vi "GetGlobalDefaultConfiguration.vi"(3 "Read defaults?":bool) -> ()   [LabVIEW 2018]
uses:
  QC_MeasurementSetup.vi
  InstrControl/InstrumentSetup.vi
  InstrControl/InstrControl.lvclass
panel:
  out "Configuration File Striptest":path
  out "Configuration File Cis":path
  out "Configuration File Stability":path
  out "Configuration File CV":path
  out "Configuration File IV":path
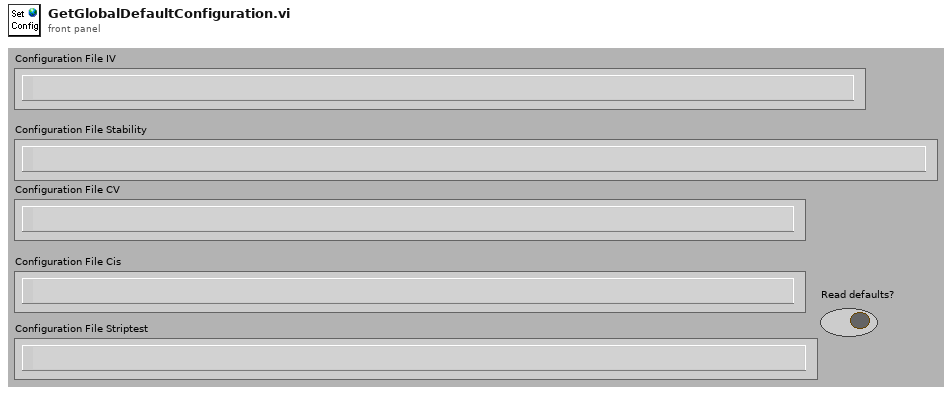
[diagram p1: front panel]
types:
  T1 = cluster{"Supply":refnum<class "SupplyControl.lvclass">, "Arduino":refnum<class "ArduinoControl.lvclass">, "Measurement switch":refnum<class "Switching.lvclass">, "Initial Voltage [V]":dbl, "Final Voltage [V]":dbl, "Step Size [V]":dbl, "Step Interval [s]":i32, "Number Of Steps":u32, "Ramp down steps [V]":dbl, "Ramp down Interval [s]":i32, "hold steps":i32, "Set Current Limit?":bool, "Current Limit [µA]":dbl, "Temperature Readout":enum16{"Read Arduino", "Enter manually"}, "Supply Name":string, "V_breakdown Limit [V]":dbl, "Measurement switch used?":bool}
  T2 = cluster{"Supply":refnum<class "SupplyControl.lvclass">, "LCR":refnum<class "LCRControl.lvclass">, "Arduino":refnum<class "ArduinoControl.lvclass">, "Measurement switch":refnum<class "Switching.lvclass">, "Initial Voltage [V]":dbl, "Final Voltage [V]":dbl, "Step Size [V]":dbl, "Step Interval [s]":i32, "Number Of Steps":u32, "Ramp down steps [V]":dbl, "Ramp down Interval [s]":i32, "Set Current Limit?":bool, "Current Limit [µA]":dbl, "Temperature Readout":enum16{"Read Arduino", "Enter manually"}, "Supply Name":string, "LCR Name":string, "V_depletion Limit [V]":dbl, "Measurement switch used?":bool}
  T3 = cluster{"RC Configuration":u16, "AC amplitude [V]":dbl, "AC frequency [Hz]":i32, "HP 4284A Configurations":cluster{"Consider OC":bool, "Consider SC":bool}}
  T4 = cluster{"Supply":refnum<class "SupplyControl.lvclass">, "DMM":refnum<class "MultimeterControl.lvclass">, "DUT switch":refnum<class "Switching.lvclass">, "Arduino":refnum<class "ArduinoControl.lvclass">, "Measurement switch":refnum<class "Switching.lvclass">, "Voltage [V]":dbl, "Measurement Interval [s]":i32, "Test Duration":u32, "Ramp up steps [V]":dbl, "Ramp up Interval [s]":u32, "Ramp down steps [V]":dbl, "Ramp down Interval [s]":i32, "Set Current Limit?":bool, "Current Limit [µA]":dbl, "Temperature Readout":enum16{"Read Arduino", "Enter manually"}, "Supply Name":string, "DMM Name":string, "Maximum current fluctuation [%]":dbl, "Measurement switch used?":bool, "DUT switch used?":bool}
  T5 = cluster{"Supply":refnum<class "SupplyControl.lvclass">, "LCR":refnum<class "LCRControl.lvclass">, "Arduino":refnum<class "ArduinoControl.lvclass">, "Measurement switch":refnum<class "Switching.lvclass">, "Initial Voltage [V]":dbl, "Final Voltage [V]":dbl, "Step Size [V]":dbl, "Step Interval [s]":i32, "Number Of Steps":u32, "AC frequency [Hz]":i32, "RC Configuration":u16, "AC amplitude [V]":dbl, "Ramp down steps [V]":dbl, "Ramp down Interval [s]":i32, "Set Current Limit?":bool, "Current Limit [µA]":dbl, "Temperature Readout":enum16{"Read Arduino", "Enter manually"}, "Supply Name":string, "LCR Name":string, "C_is Limit [pF/cm]":dbl, "Measurement switch used?":bool}
  T6 = cluster{"Bias Supply":refnum<class "SupplyControl.lvclass">, "SMU":refnum<class "SupplyControl.lvclass">, "LCR":refnum<class "LCRControl.lvclass">, "ProbeStation":refnum<class "ProbeStationControl.lvclass">, "Arduino":refnum<class "ArduinoControl.lvclass">, "Measurement switch":refnum<class "Switching.lvclass">, "Probe Card Channels":i32, "Bias Voltage [V]":dbl, "First strip":i32, "Last strip":i32, "Base Voltage [V]":dbl, "Base Ramp Step [V]":dbl, "Base Ramp Interval [ms]":u32, "High Voltage [V]":dbl, "High Ramp Step [V]":dbl, "High Ramp Interval [ms]":u32, "AC frequency [Hz]":i32, "AC amplitude [V]":dbl, "RC Configuration":u16, "Single Needle":bool, "Temperature Readout":enum16{"Read Arduino", "Enter manually"}, "Fraction of good strips [%]":dbl, "Measurement switch used?":bool, "Matrix X Channels":cluster{"Mux1 C1":i32, "Mux1 C2":i32, "Mux2 C1":i32, "Mux2 C2":i32}, "Pinholes Y/N":bool, "Capacitance Y/N":bool, "Resistance Y/N":bool, "Bias Supply Name":string, "SMU Name":string, "LCR Name":string}
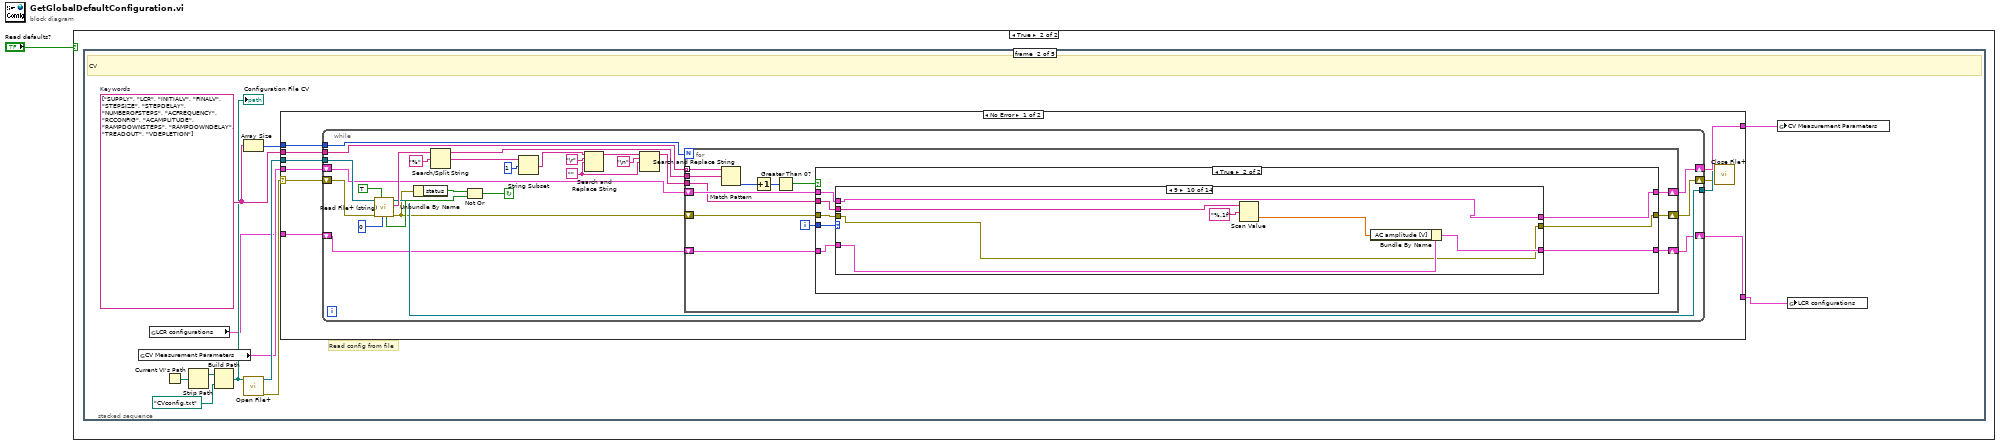
[diagram p0: block diagram]
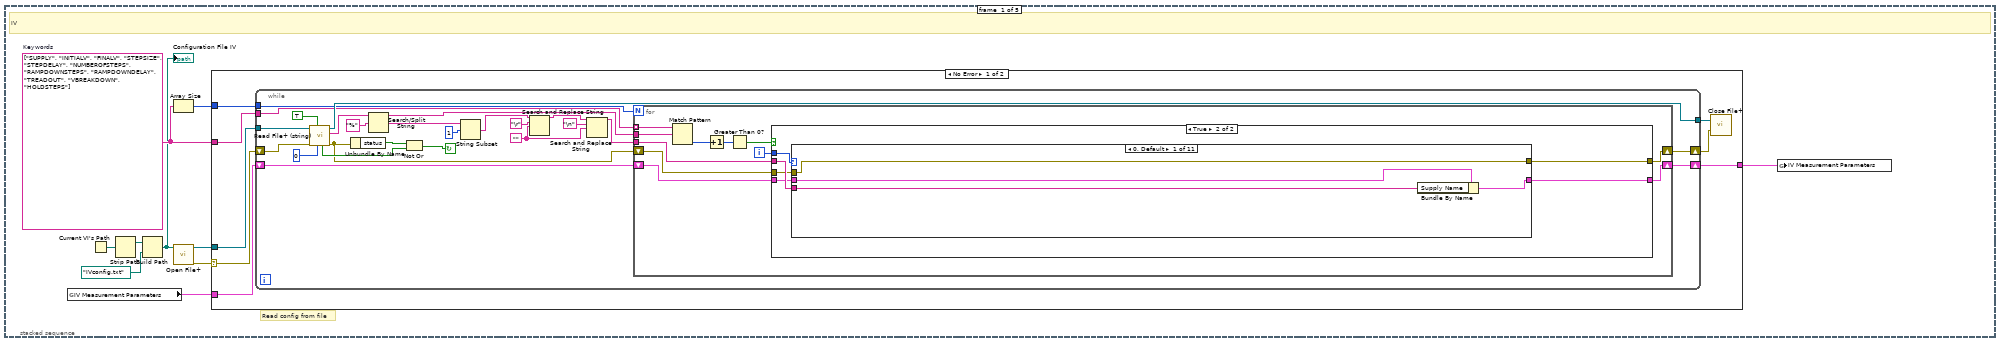
[diagram p3: hidden frame]
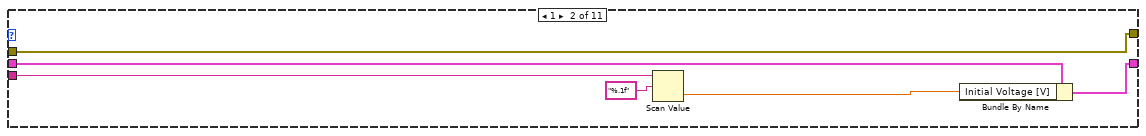
[diagram p5: hidden frame]
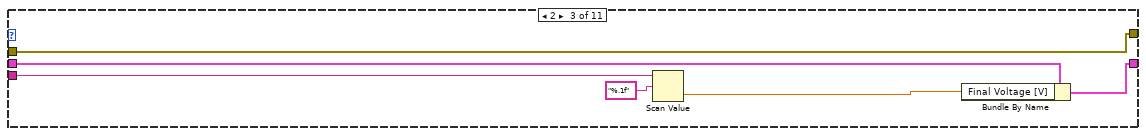
[diagram p6: hidden frame]
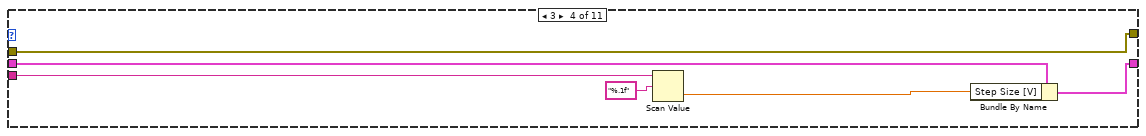
[diagram p7: hidden frame]
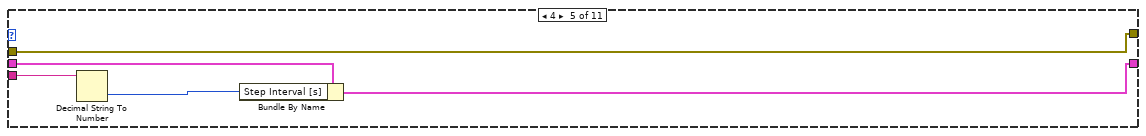
[diagram p8: hidden frame]
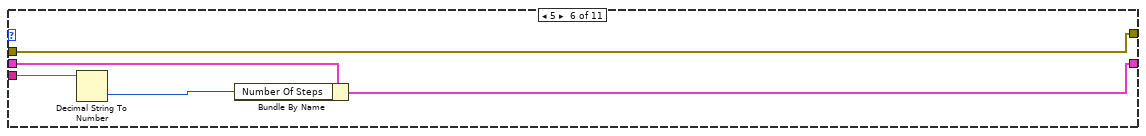
[diagram p9: hidden frame]
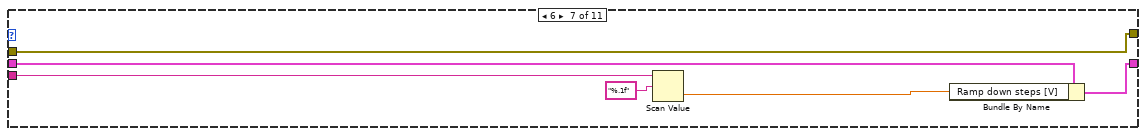
[diagram p10: hidden frame]
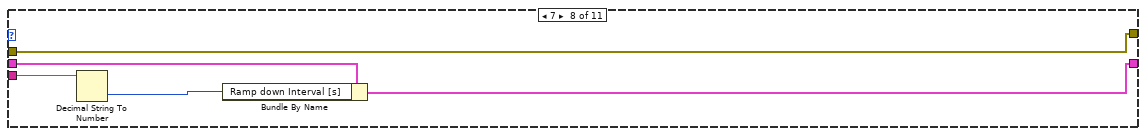
[diagram p11: hidden frame]
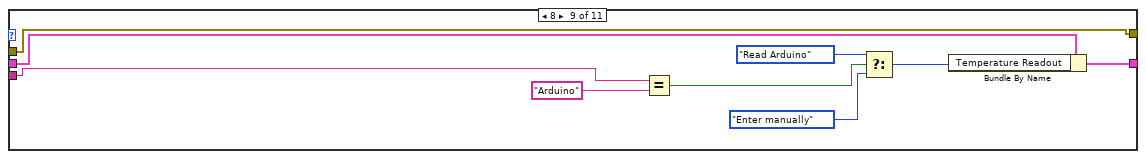
[diagram p12: hidden frame]
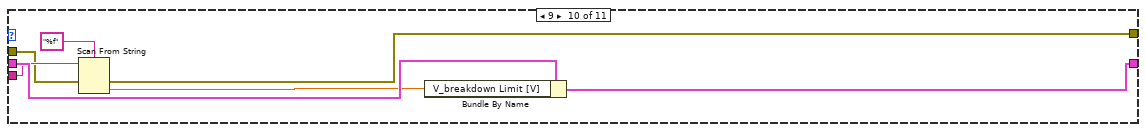
[diagram p13: hidden frame]
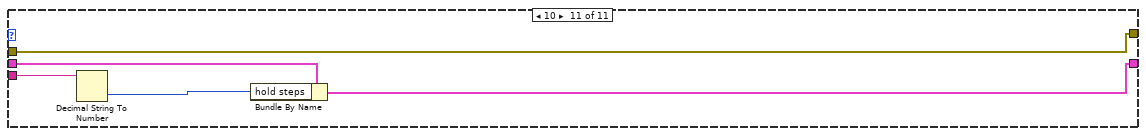
[diagram p14: hidden frame]
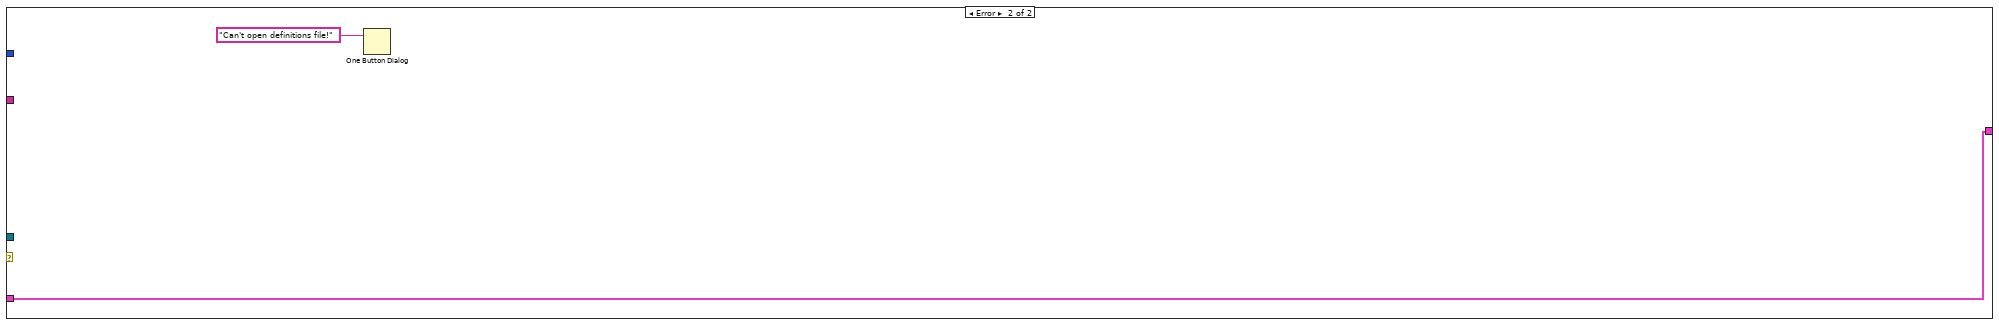
[diagram p15: hidden frame]
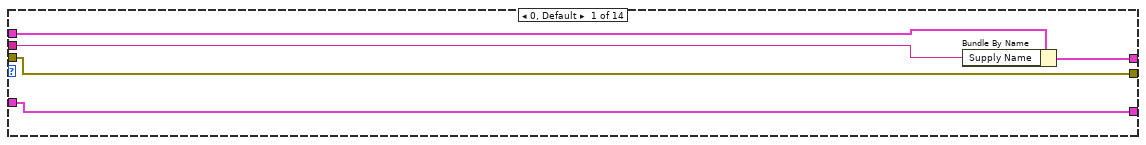
[diagram p17: hidden frame]
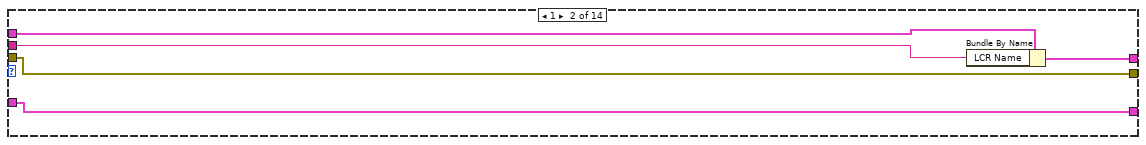
[diagram p18: hidden frame]
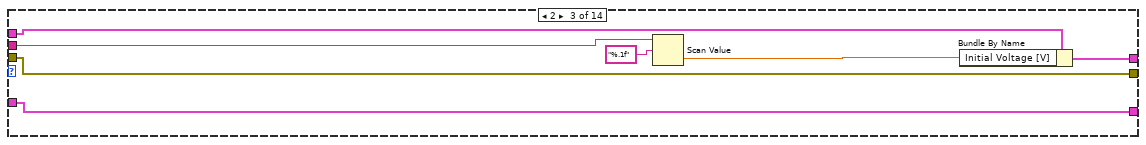
[diagram p19: hidden frame]
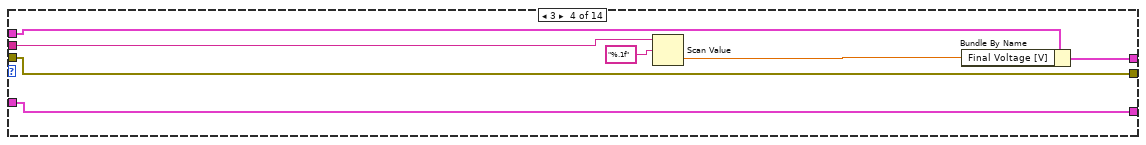
[diagram p20: hidden frame]
diagram:
  n1 = case shown="True" "Read defaults?" {
    frame False {
    }
    frame True {
      n2 = stacked-sequence {
        frame #0 {
          w11 = string[] ["SUPPLY", "INITIALV", "FINALV", "STEPSIZE", "STEPDELAY", "NUMBEROFSTEPS", "RAMPDOWNSTEPS", "RAMPDOWNDELAY", "TREADOUT", "VBREAKDOWN", "HOLDSTEPS"]  # Keywords
          # "Read config from file"
          # "IV"
          n3 = global read "QC_MeasurementSetup.vi" "IV Measurement Parameters"() -> (w2:T1)
          n4 = Current VI's Path() -> (path=w6:path)
          n5 = Strip Path(path=w6) -> (stripped path=w5:path)  [unwired: 1 out]
          n6 = Build Path(base path=w5, name or relative path=path "IVconfig.txt") -> (appended path=w4:path)
          "Configuration File IV" <- w4
          n7 = Array Size(array=w11) -> (size(s)=w10:i32)
          n8 = call <vilib>:"Open File+.vi"("file path (\" \")"=w4) -> ("error out"=w7:errorcluster, "refnum"=w8:refnum<file>)  [unwired: 7 in, 2 out]
          n9 = case shown="No Error" w7 {
            selector: w7 -> [w12 _]
            tunnel: w8 -> [w19 _]
            tunnel: w11 -> [w18 _]
            tunnel: w10 -> [w17 _]
            tunnel: w2 -> [w16 w128]
            tunnel: [w15 w128] -> w3
            frame No Error {
              n10 = while {
                shift-left: w16 -> [w30]
                shift-right: [w29] -> w15
                tunnel: w17 -> [w28]
                tunnel: w18 -> [w32]
                tunnel: [w35] -> w14
                tunnel: w19 -> [w41]
                shift-right: [w26] -> w13
                shift-left: w12 -> [w34]
                stop <- w37 continue-if-true
                w23 = ""
                n11 = call <vilib>:"Read File+ (string).vi"("count"=0, "line mode (characters:F)"=TRUE, "error in (no error)"=w34, "refnum"=w41) -> ("error out"=w27:errorcluster, "string"=w36:string, "dup refnum"=w35:refnum<file>, "EOF?"=w39:bool)  [unwired: 3 in, 1 out]
                n12 = Unbundle By Name(w27) -> ("status"=w38:bool)
                n13 = Search/Split String(string=w36, search string/char (-)="%" ("search char (-)")) -> (substring before match=w31:string, match + rest of string=w42:string)  [unwired: 1 in, 1 out]
                n14 = Not Or(1:w39, 2:w38) -> (0:w37:bool)
                n15 = String Subset(string=w42, offset (0)=1) -> (substring=w21:string)  [unwired: 1 in]
                n16 = Search and Replace String(input string=w21, search string="\r", replace string=w23) -> (result string=w22:string)  [unwired: 5 in, 3 out]
                n17 = Search and Replace String(input string=w22, search string="\n", replace string=w23) -> (result string=w20:string)  [unwired: 5 in, 3 out]
                n18 = for {
                  N: w28 -> [_]
                  tunnel: w32 -> [w53] mode=indexing
                  tunnel: w31 -> [w48]
                  shift-right: [w49] -> w29
                  shift-left: w30 -> [w50]
                  tunnel: w20 -> [w47]
                  shift-right: [w45] -> w26
                  shift-left: w27 -> [w46]
                  i -> [w51]
                  n19 = Match Pattern(string=w53, regular expression=w48) -> (offset past match=w54:i32)  [unwired: 1 in, 3 out]
                  n20 = Increment(x=w54) -> (x+1=w55:i32)
                  n21 = Greater Than 0?(x=w55) -> (x > 0?=w52:bool)
                  n22 = case shown="True" w52 {
                    tunnel: w51 -> [_ w63]
                    tunnel: w47 -> [_ w62]
                    tunnel: w50 -> [w57 w61]
                    tunnel: [w57 w60] -> w49
                    tunnel: w46 -> [w56 w59]
                    tunnel: [w56 w58] -> w45
                    frame False {
                    }
                    frame True {
                      n23 = case shown="0, Default" w63 {
                        tunnel: w62 -> [w65 w71 w76 w82 w88 w93 w98 w104 w113 w120 w124]
                        tunnel: w61 -> [w66 w73 w79 w85 w90 w95 w101 w106 w115 w122 w127]
                        tunnel: [w67 w72 w78 w84 w89 w94 w100 w105 w114 w121 w126] -> w60
                        tunnel: w59 -> [w64 w68 w74 w80 w86 w91 w96 w102 w112 w117 w123]
                        tunnel: [w64 w68 w74 w80 w86 w91 w96 w102 w112 w116 w123] -> w58
                        frame 0, Default {
                          n24 = Bundle By Name(cluster=w66, "Supply Name"=w65) -> (w67:T1)
                        }
                        frame 1 {
                          n25 = Scan Value(string=w71, format string="%.1f") -> (value=w70:dbl)  [unwired: 1 in, 1 out]
                          n26 = Bundle By Name(cluster=w73, "Initial Voltage [V]"=w70) -> (w72:T1)
                        }
                        frame 2 {
                          n27 = Scan Value(string=w76, format string="%.1f") -> (value=w75:dbl)  [unwired: 1 in, 1 out]
                          n28 = Bundle By Name(cluster=w79, "Final Voltage [V]"=w75) -> (w78:T1)
                        }
                        frame 3 {
                          n29 = Scan Value(string=w82, format string="%.1f") -> (value=w81:dbl)  [unwired: 1 in, 1 out]
                          n30 = Bundle By Name(cluster=w85, "Step Size [V]"=w81) -> (w84:T1)
                        }
                        frame 4 {
                          n31 = Decimal String To Number(string=w88) -> (number=w87:i32)  [unwired: 2 in, 1 out]
                          n32 = Bundle By Name(cluster=w90, "Step Interval [s]"=w87) -> (w89:T1)
                        }
                        frame 5 {
                          n33 = Decimal String To Number(string=w93) -> (number=w92:i32)  [unwired: 2 in, 1 out]
                          n34 = Bundle By Name(cluster=w95, "Number Of Steps"=w92) -> (w94:T1)
                        }
                        frame 6 {
                          n35 = Scan Value(string=w98, format string="%.1f") -> (value=w97:dbl)  [unwired: 1 in, 1 out]
                          n36 = Bundle By Name(cluster=w101, "Ramp down steps [V]"=w97) -> (w100:T1)
                        }
                        frame 7 {
                          n37 = Decimal String To Number(string=w104) -> (number=w103:i32)  [unwired: 2 in, 1 out]
                          n38 = Bundle By Name(cluster=w106, "Ramp down Interval [s]"=w103) -> (w105:T1)
                        }
                        frame 8 {
                          n39 = Equal?(x=w113, y="Arduino") -> (x = y?=w110:bool)
                          n40 = Select(t=enum16{"Read Arduino", "Enter manually"}."Read Arduino" ("Temperature Readout"), s=w110, f=enum16{"Read Arduino", "Enter manually"}."Enter manually" ("Temperature Readout")) -> (s? t:f=w107:enum16{"Read Arduino", "Enter manually"})
                          n41 = Bundle By Name(cluster=w115, "Temperature Readout"=w107) -> (w114:T1)
                        }
                        frame 9 {
                          n42 = Scan From String(format string="%f", input string=w120, error in=w117) -> (error out=w116:errorcluster, output 1=w119:dbl)  [unwired: 2 in, 2 out]
                          n43 = Bundle By Name(cluster=w122, "V_breakdown Limit [V]"=w119) -> (w121:T1)
                        }
                        frame 10 {
                          n44 = Decimal String To Number(string=w124) -> (number=w125:i32)  [unwired: 2 in, 1 out]
                          n45 = Bundle By Name(cluster=w127, "hold steps"=w125) -> (w126:T1)
                        }
                      }
                    }
                  }
                }
              }
              n46 = call <vilib>:"Close File+.vi"("error in (no error)"=w13, "refnum"=w14) -> ()  [unwired: 3 in, 3 out]
            }
            frame Error {
              n47 = One Button Dialog(message="Can't open definitions file!") -> ()  [unwired: 1 in, 1 out]
            }
          }
          n48 = global write "QC_MeasurementSetup.vi" "IV Measurement Parameters"(w3) -> ()
        }
        frame #1 {
          w141 = string[] ["SUPPLY", "LCR", "INITIALV", "FINALV", "STEPSIZE", "STEPDELAY", "NUMBEROFSTEPS", "ACFREQUENCY", "RCCONFIG", "ACAMPLITUDE", "RAMPDOWNSTEPS", "RAMPDOWNDELAY", "TREADOUT", "VDEPLETION"]  # Keywords
          # "Read config from file"
          # "CV"
          n49 = global read "QC_MeasurementSetup.vi" "CV Measurement Parameters"() -> (w132:T2)
          n50 = global read "InstrumentSetup.vi" "LCR configurations"() -> (w131:T3)
          n51 = Current VI's Path() -> (path=w136:path)
          n52 = Strip Path(path=w136) -> (stripped path=w135:path)  [unwired: 1 out]
          n53 = Build Path(base path=w135, name or relative path=path "CVconfig.txt") -> (appended path=w134:path)
          "Configuration File CV" <- w134
          n54 = Array Size(array=w141) -> (size(s)=w140:i32)
          n55 = call <vilib>:"Open File+.vi"("file path (\" \")"=w134) -> ("error out"=w137:errorcluster, "refnum"=w138:refnum<file>)  [unwired: 7 in, 2 out]
          n56 = case shown="No Error" w137 {
            selector: w137 -> [w144 _]
            tunnel: w138 -> [w151 _]
            tunnel: w141 -> [w150 _]
            tunnel: w140 -> [w149 _]
            tunnel: w132 -> [w148 w301]
            tunnel: [w147 w301] -> w133
            tunnel: w131 -> [w142 w300]
            tunnel: [w143 w300] -> w130
            frame No Error {
              n57 = while {
                shift-left: w148 -> [w164]
                shift-right: [w163] -> w147
                tunnel: w149 -> [w162]
                tunnel: w150 -> [w166]
                tunnel: [w169] -> w146
                tunnel: w151 -> [w175]
                shift-right: [w160] -> w145
                shift-left: w144 -> [w168]
                shift-right: [w153] -> w143
                shift-left: w142 -> [w152]
                stop <- w171 continue-if-true
                w157 = ""
                n58 = call <vilib>:"Read File+ (string).vi"("count"=0, "line mode (characters:F)"=TRUE, "error in (no error)"=w168, "refnum"=w175) -> ("error out"=w161:errorcluster, "string"=w170:string, "dup refnum"=w169:refnum<file>, "EOF?"=w173:bool)  [unwired: 3 in, 1 out]
                n59 = Unbundle By Name(w161) -> ("status"=w172:bool)
                n60 = Search/Split String(string=w170, search string/char (-)="%" ("search char (-)")) -> (substring before match=w165:string, match + rest of string=w176:string)  [unwired: 1 in, 1 out]
                n61 = Not Or(1:w173, 2:w172) -> (0:w171:bool)
                n62 = String Subset(string=w176, offset (0)=1) -> (substring=w155:string)  [unwired: 1 in]
                n63 = Search and Replace String(input string=w155, search string="\r", replace string=w157) -> (result string=w156:string)  [unwired: 5 in, 3 out]
                n64 = Search and Replace String(input string=w156, search string="\n", replace string=w157) -> (result string=w154:string)  [unwired: 5 in, 3 out]
                n65 = for {
                  N: w162 -> [_]
                  tunnel: w166 -> [w189] mode=indexing
                  tunnel: w165 -> [w184]
                  shift-right: [w185] -> w163
                  shift-left: w164 -> [w186]
                  tunnel: w154 -> [w183]
                  shift-right: [w181] -> w160
                  shift-left: w161 -> [w182]
                  shift-right: [w179] -> w153
                  shift-left: w152 -> [w180]
                  i -> [w187]
                  n66 = Match Pattern(string=w189, regular expression=w184) -> (offset past match=w190:i32)  [unwired: 1 in, 3 out]
                  n67 = Increment(x=w190) -> (x+1=w191:i32)
                  n68 = Greater Than 0?(x=w191) -> (x > 0?=w188:bool)
                  n69 = case shown="True" w188 {
                    tunnel: w187 -> [_ w202]
                    tunnel: w183 -> [_ w201]
                    tunnel: w186 -> [w194 w200]
                    tunnel: [w194 w199] -> w185
                    tunnel: w182 -> [w193 w198]
                    tunnel: [w193 w197] -> w181
                    tunnel: [w192 w195] -> w179
                    tunnel: w180 -> [w192 w196]
                    frame False {
                    }
                    frame True {
                      n70 = case shown="9" w202 {
                        tunnel: w201 -> [w205 w210 w217 w223 w230 w237 w243 w251 w260 w268 w272 w279 w289 w297]
                        tunnel: w200 -> [w206 w211 w219 w226 w233 w239 w245 w246 w252 w262 w275 w281 w291 w293]
                        tunnel: [w207 w212 w218 w225 w232 w238 w244 w246 w252 w262 w274 w280 w290 w294] -> w199
                        tunnel: w198 -> [w204 w209 w214 w221 w228 w235 w241 w247 w253 w263 w270 w277 w288 w296]
                        tunnel: [w204 w209 w214 w221 w228 w235 w241 w247 w253 w263 w270 w277 w288 w295] -> w197
                        tunnel: w196 -> [w203 w208 w213 w220 w227 w234 w240 w250 w256 w266 w269 w276 w282 w292]
                        tunnel: [w203 w208 w213 w220 w227 w234 w240 w248 w254 w264 w269 w276 w282 w292] -> w195
                        frame 0, Default {
                          n71 = Bundle By Name(cluster=w206, "Supply Name"=w205) -> (w207:T2)
                        }
                        frame 1 {
                          n72 = Bundle By Name(cluster=w211, "LCR Name"=w210) -> (w212:T2)
                        }
                        frame 2 {
                          n73 = Scan Value(string=w217, format string="%.1f") -> (value=w216:dbl)  [unwired: 1 in, 1 out]
                          n74 = Bundle By Name(cluster=w219, "Initial Voltage [V]"=w216) -> (w218:T2)
                        }
                        frame 3 {
                          n75 = Scan Value(string=w223, format string="%.1f") -> (value=w222:dbl)  [unwired: 1 in, 1 out]
                          n76 = Bundle By Name(cluster=w226, "Final Voltage [V]"=w222) -> (w225:T2)
                        }
                        frame 4 {
                          n77 = Scan Value(string=w230, format string="%.1f") -> (value=w229:dbl)  [unwired: 1 in, 1 out]
                          n78 = Bundle By Name(cluster=w233, "Step Size [V]"=w229) -> (w232:T2)
                        }
                        frame 5 {
                          n79 = Decimal String To Number(string=w237) -> (number=w236:i32)  [unwired: 2 in, 1 out]
                          n80 = Bundle By Name(cluster=w239, "Step Interval [s]"=w236) -> (w238:T2)
                        }
                        frame 6 {
                          n81 = Decimal String To Number(string=w243) -> (number=w242:i32)  [unwired: 2 in, 1 out]
                          n82 = Bundle By Name(cluster=w245, "Number Of Steps"=w242) -> (w244:T2)
                        }
                        frame 7 {
                          n83 = Decimal String To Number(string=w251) -> (number=w249:i32)  [unwired: 2 in, 1 out]
                          n84 = Bundle By Name(cluster=w250, "AC frequency [Hz]"=w249) -> (w248:T3)
                        }
                        frame 8 {
                          w259 = u16 0 items=["serial", "parallel"] ("RC Configuration")
                          w258 = u16 1 items=["serial", "parallel"] ("RC Configuration")
                          n85 = Equal?(x=w260, y="serial") -> (x = y?=w257:bool)
                          n86 = Select(t=w259, s=w257, f=w258) -> (s? t:f=w255:u16)
                          n87 = Bundle By Name(cluster=w256, "RC Configuration"=w255) -> (w254:T3)
                        }
                        frame 9 {
                          n88 = Scan Value(string=w268, format string="%.1f") -> (value=w265:dbl)  [unwired: 1 in, 1 out]
                          n89 = Bundle By Name(cluster=w266, "AC amplitude [V]"=w265) -> (w264:T3)
                        }
                        frame 10 {
                          n90 = Scan Value(string=w272, format string="%.1f") -> (value=w271:dbl)  [unwired: 1 in, 1 out]
                          n91 = Bundle By Name(cluster=w275, "Ramp down steps [V]"=w271) -> (w274:T2)
                        }
                        frame 11 {
                          n92 = Decimal String To Number(string=w279) -> (number=w278:i32)  [unwired: 2 in, 1 out]
                          n93 = Bundle By Name(cluster=w281, "Ramp down Interval [s]"=w278) -> (w280:T2)
                        }
                        frame 12 {
                          n94 = Equal?(x=w289, y="Arduino") -> (x = y?=w286:bool)
                          n95 = Select(t=enum16{"Read Arduino", "Enter manually"}."Read Arduino" ("Temperature Readout"), s=w286, f=enum16{"Read Arduino", "Enter manually"}."Enter manually" ("Temperature Readout")) -> (s? t:f=w283:enum16{"Read Arduino", "Enter manually"})
                          n96 = Bundle By Name(cluster=w291, "Temperature Readout"=w283) -> (w290:T2)
                        }
                        frame 13 {
                          n97 = Scan From String(format string="%f", input string=w297, error in=w296) -> (error out=w295:errorcluster, output 1=w299:dbl)  [unwired: 2 in, 2 out]
                          n98 = Bundle By Name(cluster=w293, "V_depletion Limit [V]"=w299) -> (w294:T2)
                        }
                      }
                    }
                  }
                }
              }
              n99 = call <vilib>:"Close File+.vi"("error in (no error)"=w145, "refnum"=w146) -> ()  [unwired: 3 in, 3 out]
            }
            frame Error {
              n100 = One Button Dialog(message="Can't open definitions file!") -> ()  [unwired: 1 in, 1 out]
            }
          }
          n101 = global write "QC_MeasurementSetup.vi" "CV Measurement Parameters"(w133) -> ()
          n102 = global write "InstrumentSetup.vi" "LCR configurations"(w130) -> ()
        }
        frame #2 {
          w312 = string[] ["SUPPLY", "DMM", "VOLTAGE", "INTERVAL", "DURATION", "RAMPUPSTEPS", "RAMPUPDELAY", "RAMPDOWNSTEPS", "RAMPDOWNDELAY", "TREADOUT", "IFLUCTUATIONS"]  # Keywords
          # "Read config from file"
          # "STABILITY"
          n103 = global read "QC_MeasurementSetup.vi" "Current Stability Measurement Parameters"() -> (w303:T4)
          n104 = Current VI's Path() -> (path=w307:path)
          n105 = Strip Path(path=w307) -> (stripped path=w306:path)  [unwired: 1 out]
          n106 = Build Path(base path=w306, name or relative path=path "STABILITYconfig.txt") -> (appended path=w305:path)
          "Configuration File Stability" <- w305
          n107 = Array Size(array=w312) -> (size(s)=w311:i32)
          n108 = call <vilib>:"Open File+.vi"("file path (\" \")"=w305) -> ("error out"=w308:errorcluster, "refnum"=w309:refnum<file>)  [unwired: 7 in, 2 out]
          n109 = case shown="No Error" w308 {
            selector: w308 -> [w313 _]
            tunnel: w309 -> [w320 _]
            tunnel: w312 -> [w319 _]
            tunnel: w311 -> [w318 _]
            tunnel: w303 -> [w317 w427]
            tunnel: [w316 w427] -> w304
            frame No Error {
              n110 = while {
                shift-left: w317 -> [w331]
                shift-right: [w330] -> w316
                tunnel: w318 -> [w329]
                tunnel: w319 -> [w333]
                tunnel: [w336] -> w315
                tunnel: w320 -> [w342]
                shift-right: [w327] -> w314
                shift-left: w313 -> [w335]
                stop <- w338 continue-if-true
                w324 = ""
                n111 = call <vilib>:"Read File+ (string).vi"("count"=0, "line mode (characters:F)"=TRUE, "error in (no error)"=w335, "refnum"=w342) -> ("error out"=w328:errorcluster, "string"=w337:string, "dup refnum"=w336:refnum<file>, "EOF?"=w340:bool)  [unwired: 3 in, 1 out]
                n112 = Unbundle By Name(w328) -> ("status"=w339:bool)
                n113 = Search/Split String(string=w337, search string/char (-)="%" ("search char (-)")) -> (substring before match=w332:string, match + rest of string=w343:string)  [unwired: 1 in, 1 out]
                n114 = Not Or(1:w340, 2:w339) -> (0:w338:bool)
                n115 = String Subset(string=w343, offset (0)=1) -> (substring=w322:string)  [unwired: 1 in]
                n116 = Search and Replace String(input string=w322, search string="\r", replace string=w324) -> (result string=w323:string)  [unwired: 5 in, 3 out]
                n117 = Search and Replace String(input string=w323, search string="\n", replace string=w324) -> (result string=w321:string)  [unwired: 5 in, 3 out]
                n118 = for {
                  N: w329 -> [_]
                  tunnel: w333 -> [w354] mode=indexing
                  tunnel: w332 -> [w349]
                  shift-right: [w350] -> w330
                  shift-left: w331 -> [w351]
                  tunnel: w321 -> [w348]
                  shift-right: [w346] -> w327
                  shift-left: w328 -> [w347]
                  i -> [w352]
                  n119 = Match Pattern(string=w354, regular expression=w349) -> (offset past match=w355:i32)  [unwired: 1 in, 3 out]
                  n120 = Increment(x=w355) -> (x+1=w356:i32)
                  n121 = Greater Than 0?(x=w356) -> (x > 0?=w353:bool)
                  n122 = case shown="True" w353 {
                    tunnel: w352 -> [_ w364]
                    tunnel: w348 -> [_ w363]
                    tunnel: w351 -> [w358 w362]
                    tunnel: [w358 w361] -> w350
                    tunnel: w347 -> [w357 w360]
                    tunnel: [w357 w359] -> w346
                    frame False {
                    }
                    frame True {
                      n123 = case shown="10" w364 {
                        tunnel: w363 -> [w365 w369 w376 w380 w385 w391 w397 w402 w408 w417 w423]
                        tunnel: w362 -> [w367 w371 w378 w383 w388 w394 w399 w405 w410 w419 w424]
                        tunnel: [w368 w372 w377 w382 w387 w393 w398 w404 w409 w418 w422] -> w361
                        tunnel: w360 -> [w366 w370 w373 w381 w386 w392 w395 w400 w406 w416 w420]
                        tunnel: [w366 w370 w373 w381 w386 w392 w395 w400 w406 w416 w421] -> w359
                        frame 0, Default {
                          n124 = Bundle By Name(cluster=w367, "Supply Name"=w365) -> (w368:T4)
                        }
                        frame 1 {
                          n125 = Bundle By Name(cluster=w371, "DMM Name"=w369) -> (w372:T4)
                        }
                        frame 2 {
                          n126 = Scan Value(string=w376, format string="%.1f") -> (value=w375:dbl)  [unwired: 1 in, 1 out]
                          n127 = Bundle By Name(cluster=w378, "Voltage [V]"=w375) -> (w377:T4)
                        }
                        frame 3 {
                          n128 = Decimal String To Number(string=w380) -> (number=w379:i32)  [unwired: 2 in, 1 out]
                          n129 = Bundle By Name(cluster=w383, "Measurement Interval [s]"=w379) -> (w382:T4)
                        }
                        frame 4 {
                          n130 = Decimal String To Number(string=w385) -> (number=w384:i32)  [unwired: 2 in, 1 out]
                          n131 = Bundle By Name(cluster=w388, "Test Duration"=w384) -> (w387:T4)
                        }
                        frame 5 {
                          n132 = Scan Value(string=w391, format string="%.1f") -> (value=w389:dbl)  [unwired: 1 in, 1 out]
                          n133 = Bundle By Name(cluster=w394, "Ramp up steps [V]"=w389) -> (w393:T4)
                        }
                        frame 6 {
                          n134 = Decimal String To Number(string=w397) -> (number=w396:i32)  [unwired: 2 in, 1 out]
                          n135 = Bundle By Name(cluster=w399, "Ramp up Interval [s]"=w396) -> (w398:T4)
                        }
                        frame 7 {
                          n136 = Scan Value(string=w402, format string="%.1f") -> (value=w401:dbl)  [unwired: 1 in, 1 out]
                          n137 = Bundle By Name(cluster=w405, "Ramp down steps [V]"=w401) -> (w404:T4)
                        }
                        frame 8 {
                          n138 = Decimal String To Number(string=w408) -> (number=w407:i32)  [unwired: 2 in, 1 out]
                          n139 = Bundle By Name(cluster=w410, "Ramp down Interval [s]"=w407) -> (w409:T4)
                        }
                        frame 9 {
                          n140 = Equal?(x=w417, y="Arduino") -> (x = y?=w414:bool)
                          n141 = Select(t=enum16{"Read Arduino", "Enter manually"}."Read Arduino" ("Temperature Readout"), s=w414, f=enum16{"Read Arduino", "Enter manually"}."Enter manually" ("Temperature Readout")) -> (s? t:f=w411:enum16{"Read Arduino", "Enter manually"})
                          n142 = Bundle By Name(cluster=w419, "Temperature Readout"=w411) -> (w418:T4)
                        }
                        frame 10 {
                          n143 = Scan From String(format string="%f", input string=w423, error in=w420) -> (error out=w421:errorcluster, output 1=w426:dbl)  [unwired: 2 in, 2 out]
                          n144 = Bundle By Name(cluster=w424, "Maximum current fluctuation [%]"=w426) -> (w422:T4)
                        }
                      }
                    }
                  }
                }
              }
              n145 = call <vilib>:"Close File+.vi"("error in (no error)"=w314, "refnum"=w315) -> ()  [unwired: 3 in, 3 out]
            }
            frame Error {
              n146 = One Button Dialog(message="Can't open definitions file!") -> ()  [unwired: 1 in, 1 out]
            }
          }
          n147 = global write "QC_MeasurementSetup.vi" "Current Stability Measurement Parameters"(w304) -> ()
        }
        frame #3 {
          w438 = string[] ["SUPPLY", "LCR", "INITIALV", "FINALV", "STEPSIZE", "STEPDELAY", "NUMBEROFSTEPS", "ACFREQUENCY", "RCCONFIG", "ACAMPLITUDE", "RAMPDOWNSTEPS", "RAMPDOWNDELAY", "TREADOUT", "CISLIMIT"]  # Keywords
          # "Read config from file"
          # "CIS"
          n148 = global read "QC_MeasurementSetup.vi" "Cis Measurement Parameters"() -> (w429:T5)
          n149 = Current VI's Path() -> (path=w433:path)
          n150 = Strip Path(path=w433) -> (stripped path=w432:path)  [unwired: 1 out]
          n151 = Build Path(base path=w432, name or relative path=path "CISconfig.txt") -> (appended path=w431:path)
          "Configuration File Cis" <- w431
          n152 = Array Size(array=w438) -> (size(s)=w437:i32)
          n153 = call <vilib>:"Open File+.vi"("file path (\" \")"=w431) -> ("error out"=w434:errorcluster, "refnum"=w435:refnum<file>)  [unwired: 7 in, 2 out]
          n154 = case shown="No Error" w434 {
            selector: w434 -> [w439 _]
            tunnel: w435 -> [w446 _]
            tunnel: w438 -> [w445 _]
            tunnel: w437 -> [w444 _]
            tunnel: w429 -> [w443 w574]
            tunnel: [w442 w574] -> w430
            frame No Error {
              n155 = while {
                shift-left: w443 -> [w457]
                shift-right: [w456] -> w442
                tunnel: w444 -> [w455]
                tunnel: w445 -> [w459]
                tunnel: [w462] -> w441
                tunnel: w446 -> [w468]
                shift-right: [w453] -> w440
                shift-left: w439 -> [w461]
                stop <- w464 continue-if-true
                w450 = ""
                n156 = call <vilib>:"Read File+ (string).vi"("count"=0, "line mode (characters:F)"=TRUE, "error in (no error)"=w461, "refnum"=w468) -> ("error out"=w454:errorcluster, "string"=w463:string, "dup refnum"=w462:refnum<file>, "EOF?"=w466:bool)  [unwired: 3 in, 1 out]
                n157 = Unbundle By Name(w454) -> ("status"=w465:bool)
                n158 = Search/Split String(string=w463, search string/char (-)="%" ("search char (-)")) -> (substring before match=w458:string, match + rest of string=w469:string)  [unwired: 1 in, 1 out]
                n159 = Not Or(1:w466, 2:w465) -> (0:w464:bool)
                n160 = String Subset(string=w469, offset (0)=1) -> (substring=w448:string)  [unwired: 1 in]
                n161 = Search and Replace String(input string=w448, search string="\r", replace string=w450) -> (result string=w449:string)  [unwired: 5 in, 3 out]
                n162 = Search and Replace String(input string=w449, search string="\n", replace string=w450) -> (result string=w447:string)  [unwired: 5 in, 3 out]
                n163 = for {
                  N: w455 -> [_]
                  tunnel: w459 -> [w480] mode=indexing
                  tunnel: w458 -> [w475]
                  shift-right: [w476] -> w456
                  shift-left: w457 -> [w477]
                  tunnel: w447 -> [w474]
                  shift-right: [w472] -> w453
                  shift-left: w454 -> [w473]
                  i -> [w478]
                  n164 = Match Pattern(string=w480, regular expression=w475) -> (offset past match=w481:i32)  [unwired: 1 in, 3 out]
                  n165 = Increment(x=w481) -> (x+1=w482:i32)
                  n166 = Greater Than 0?(x=w482) -> (x > 0?=w479:bool)
                  n167 = case shown="True" w479 {
                    tunnel: w478 -> [_ w490]
                    tunnel: w474 -> [_ w489]
                    tunnel: w477 -> [w484 w488]
                    tunnel: [w484 w487] -> w476
                    tunnel: w473 -> [w483 w486]
                    tunnel: [w483 w485] -> w472
                    frame False {
                    }
                    frame True {
                      n168 = case shown="0, Default" w490 {
                        tunnel: w489 -> [w491 w495 w502 w507 w513 w519 w524 w529 w537 w546 w549 w555 w564 w571]
                        tunnel: w488 -> [w493 w497 w504 w510 w516 w521 w526 w531 w540 w544 w552 w557 w566 w570]
                        tunnel: [w494 w498 w503 w509 w515 w520 w525 w530 w539 w542 w551 w556 w565 w569] -> w487
                        tunnel: w486 -> [w492 w496 w499 w505 w511 w517 w522 w527 w532 w541 w547 w553 w563 w567]
                        tunnel: [w492 w496 w499 w505 w511 w517 w522 w527 w532 w541 w547 w553 w563 w568] -> w485
                        frame 0, Default {
                          n169 = Bundle By Name(cluster=w493, "Supply Name"=w491) -> (w494:T5)
                        }
                        frame 1 {
                          n170 = Bundle By Name(cluster=w497, "LCR Name"=w495) -> (w498:T5)
                        }
                        frame 2 {
                          n171 = Scan Value(string=w502, format string="%.1f") -> (value=w501:dbl)  [unwired: 1 in, 1 out]
                          n172 = Bundle By Name(cluster=w504, "Initial Voltage [V]"=w501) -> (w503:T5)
                        }
                        frame 3 {
                          n173 = Scan Value(string=w507, format string="%.1f") -> (value=w506:dbl)  [unwired: 1 in, 1 out]
                          n174 = Bundle By Name(cluster=w510, "Final Voltage [V]"=w506) -> (w509:T5)
                        }
                        frame 4 {
                          n175 = Scan Value(string=w513, format string="%.1f") -> (value=w512:dbl)  [unwired: 1 in, 1 out]
                          n176 = Bundle By Name(cluster=w516, "Step Size [V]"=w512) -> (w515:T5)
                        }
                        frame 5 {
                          n177 = Decimal String To Number(string=w519) -> (number=w518:i32)  [unwired: 2 in, 1 out]
                          n178 = Bundle By Name(cluster=w521, "Step Interval [s]"=w518) -> (w520:T5)
                        }
                        frame 6 {
                          n179 = Decimal String To Number(string=w524) -> (number=w523:i32)  [unwired: 2 in, 1 out]
                          n180 = Bundle By Name(cluster=w526, "Number Of Steps"=w523) -> (w525:T5)
                        }
                        frame 7 {
                          n181 = Decimal String To Number(string=w529) -> (number=w528:i32)  [unwired: 2 in, 1 out]
                          n182 = Bundle By Name(cluster=w531, "AC frequency [Hz]"=w528) -> (w530:T5)
                        }
                        frame 8 {
                          w536 = u16 0 items=["serial", "parallel"] ("RC Configuration")
                          w535 = u16 1 items=["serial", "parallel"] ("RC Configuration")
                          n183 = Equal?(x=w537, y="serial") -> (x = y?=w534:bool)
                          n184 = Select(t=w536, s=w534, f=w535) -> (s? t:f=w533:u16)
                          n185 = Bundle By Name(cluster=w540, "RC Configuration"=w533) -> (w539:T5)
                        }
                        frame 9 {
                          n186 = Scan Value(string=w546, format string="%.1f") -> (value=w543:dbl)  [unwired: 1 in, 1 out]
                          n187 = Bundle By Name(cluster=w544, "AC amplitude [V]"=w543) -> (w542:T5)
                        }
                        frame 10 {
                          n188 = Scan Value(string=w549, format string="%.1f") -> (value=w548:dbl)  [unwired: 1 in, 1 out]
                          n189 = Bundle By Name(cluster=w552, "Ramp down steps [V]"=w548) -> (w551:T5)
                        }
                        frame 11 {
                          n190 = Decimal String To Number(string=w555) -> (number=w554:i32)  [unwired: 2 in, 1 out]
                          n191 = Bundle By Name(cluster=w557, "Ramp down Interval [s]"=w554) -> (w556:T5)
                        }
                        frame 12 {
                          n192 = Equal?(x=w564, y="Arduino") -> (x = y?=w561:bool)
                          n193 = Select(t=enum16{"Read Arduino", "Enter manually"}."Read Arduino" ("Temperature Readout"), s=w561, f=enum16{"Read Arduino", "Enter manually"}."Enter manually" ("Temperature Readout")) -> (s? t:f=w558:enum16{"Read Arduino", "Enter manually"})
                          n194 = Bundle By Name(cluster=w566, "Temperature Readout"=w558) -> (w565:T5)
                        }
                        frame 13 {
                          n195 = Scan From String(format string="%f", input string=w571, error in=w567) -> (error out=w568:errorcluster, output 1=w573:dbl)  [unwired: 2 in, 2 out]
                          n196 = Bundle By Name(cluster=w570, "C_is Limit [pF/cm]"=w573) -> (w569:T5)
                        }
                      }
                    }
                  }
                }
              }
              n197 = call <vilib>:"Close File+.vi"("error in (no error)"=w440, "refnum"=w441) -> ()  [unwired: 3 in, 3 out]
            }
            frame Error {
              n198 = One Button Dialog(message="Can't open definitions file!") -> ()  [unwired: 1 in, 1 out]
            }
          }
          n199 = global write "QC_MeasurementSetup.vi" "Cis Measurement Parameters"(w430) -> ()
        }
        frame #4 {
          w585 = string[] ["BIASSUPPLY", "SMU", "LCR", "BIASV", "BASEV", "BASERAMP", "BASEINT", "HIGHV", "HIGHRAMP", "HIGHINT", "ACFREQUENCY", "RCCONFIG", "ACAMPLITUDE", "TREADOUT", "GOODSTRIPS", "CARD"]  # Keywords
          # "Read config from file"
          # "STRIPTEST"
          n200 = global read "QC_MeasurementSetup.vi" "Striptest Measurement Parameters"() -> (w577:T6)
          n201 = Current VI's Path() -> (path=w580:path)
          n202 = Strip Path(path=w580) -> (stripped path=w579:path)  [unwired: 1 out]
          n203 = Build Path(base path=w579, name or relative path=path "STRIPTESTconfig.txt") -> (appended path=w576:path)
          "Configuration File Striptest" <- w576
          n204 = Array Size(array=w585) -> (size(s)=w584:i32)
          n205 = call <vilib>:"Open File+.vi"("file path (\" \")"=w576) -> ("error out"=w581:errorcluster, "refnum"=w582:refnum<file>)  [unwired: 7 in, 2 out]
          n206 = case shown="No Error" w581 {
            selector: w581 -> [w586 _]
            tunnel: w582 -> [w593 _]
            tunnel: w585 -> [w592 _]
            tunnel: w584 -> [w591 _]
            tunnel: w577 -> [w590 w730]
            tunnel: [w589 w730] -> w578
            frame No Error {
              n207 = while {
                shift-left: w590 -> [w604]
                shift-right: [w603] -> w589
                tunnel: w591 -> [w602]
                tunnel: w592 -> [w606]
                tunnel: [w609] -> w588
                tunnel: w593 -> [w615]
                shift-right: [w600] -> w587
                shift-left: w586 -> [w608]
                stop <- w611 continue-if-true
                w597 = ""
                n208 = call <vilib>:"Read File+ (string).vi"("count"=0, "line mode (characters:F)"=TRUE, "error in (no error)"=w608, "refnum"=w615) -> ("error out"=w601:errorcluster, "string"=w610:string, "dup refnum"=w609:refnum<file>, "EOF?"=w613:bool)  [unwired: 3 in, 1 out]
                n209 = Unbundle By Name(w601) -> ("status"=w612:bool)
                n210 = Search/Split String(string=w610, search string/char (-)="%" ("search char (-)")) -> (substring before match=w605:string, match + rest of string=w616:string)  [unwired: 1 in, 1 out]
                n211 = Not Or(1:w613, 2:w612) -> (0:w611:bool)
                n212 = String Subset(string=w616, offset (0)=1) -> (substring=w595:string)  [unwired: 1 in]
                n213 = Search and Replace String(input string=w595, search string="\r", replace string=w597) -> (result string=w596:string)  [unwired: 5 in, 3 out]
                n214 = Search and Replace String(input string=w596, search string="\n", replace string=w597) -> (result string=w594:string)  [unwired: 5 in, 3 out]
                n215 = for {
                  N: w602 -> [_]
                  tunnel: w606 -> [w627] mode=indexing
                  tunnel: w605 -> [w622]
                  shift-right: [w623] -> w603
                  shift-left: w604 -> [w624]
                  tunnel: w594 -> [w621]
                  shift-right: [w619] -> w600
                  shift-left: w601 -> [w620]
                  i -> [w625]
                  n216 = Match Pattern(string=w627, regular expression=w622) -> (offset past match=w628:i32)  [unwired: 1 in, 3 out]
                  n217 = Increment(x=w628) -> (x+1=w629:i32)
                  n218 = Greater Than 0?(x=w629) -> (x > 0?=w626:bool)
                  n219 = case shown="True" w626 {
                    tunnel: w625 -> [_ w637]
                    tunnel: w621 -> [_ w636]
                    tunnel: w624 -> [w631 w635]
                    tunnel: [w631 w634] -> w623
                    tunnel: w620 -> [w630 w633]
                    tunnel: [w630 w632] -> w619
                    frame False {
                    }
                    frame True {
                      n220 = case shown="0, Default" w637 {
                        tunnel: w636 -> [w638 w642 w647 w653 w659 w665 w669 w676 w682 w686 w691 w700 w705 w716 w722 w726]
                        tunnel: w635 -> [w640 w644 w648 w655 w661 w667 w672 w673 w679 w687 w692 w703 w708 w718 w721 w729]
                        tunnel: [w641 w645 w649 w654 w660 w666 w671 w674 w680 w688 w693 w702 w707 w717 w719 w727] -> w634
                        tunnel: w633 -> [w639 w643 w646 w650 w656 w662 w670 w675 w681 w689 w694 w695 w704 w715 w720 w728]
                        tunnel: [w639 w643 w646 w650 w656 w662 w670 w675 w681 w689 w694 w695 w704 w715 w720 w728] -> w632
                        frame 0, Default {
                          n221 = Bundle By Name(cluster=w640, "Bias Supply Name"=w638) -> (w641:T6)
                        }
                        frame 1 {
                          n222 = Bundle By Name(cluster=w644, "SMU Name"=w642) -> (w645:T6)
                        }
                        frame 2 {
                          n223 = Bundle By Name(cluster=w648, "LCR Name"=w647) -> (w649:T6)
                        }
                        frame 3 {
                          n224 = Scan Value(string=w653, format string="%.1f") -> (value=w652:dbl)  [unwired: 1 in, 1 out]
                          n225 = Bundle By Name(cluster=w655, "Bias Voltage [V]"=w652) -> (w654:T6)
                        }
                        frame 4 {
                          n226 = Scan Value(string=w659, format string="%.1f") -> (value=w658:dbl)  [unwired: 1 in, 1 out]
                          n227 = Bundle By Name(cluster=w661, "Base Voltage [V]"=w658) -> (w660:T6)
                        }
                        frame 5 {
                          n228 = Scan Value(string=w665, format string="%.1f") -> (value=w664:dbl)  [unwired: 1 in, 1 out]
                          n229 = Bundle By Name(cluster=w667, "Base Ramp Step [V]"=w664) -> (w666:T6)
                        }
                        frame 6 {
                          n230 = Decimal String To Number(string=w669) -> (number=w668:i32)  [unwired: 2 in, 1 out]
                          n231 = Bundle By Name(cluster=w672, "Base Ramp Interval [ms]"=w668) -> (w671:T6)
                        }
                        frame 7 {
                          n232 = Scan Value(string=w676, format string="%.1f") -> (value=w678:dbl)  [unwired: 1 in, 1 out]
                          n233 = Bundle By Name(cluster=w673, "High Voltage [V]"=w678) -> (w674:T6)
                        }
                        frame 8 {
                          n234 = Scan Value(string=w682, format string="%.1f") -> (value=w684:dbl)  [unwired: 1 in, 1 out]
                          n235 = Bundle By Name(cluster=w679, "High Ramp Step [V]"=w684) -> (w680:T6)
                        }
                        frame 9 {
                          n236 = Decimal String To Number(string=w686) -> (number=w685:i32)  [unwired: 2 in, 1 out]
                          n237 = Bundle By Name(cluster=w687, "High Ramp Interval [ms]"=w685) -> (w688:T6)
                        }
                        frame 10 {
                          n238 = Decimal String To Number(string=w691) -> (number=w690:i32)  [unwired: 2 in, 1 out]
                          n239 = Bundle By Name(cluster=w692, "AC frequency [Hz]"=w690) -> (w693:T6)
                        }
                        frame 11 {
                          w699 = u16 0 items=["serial", "parallel"] ("RC Configuration")
                          w698 = u16 1 items=["serial", "parallel"] ("RC Configuration")
                          n240 = Equal?(x=w700, y="serial") -> (x = y?=w697:bool)
                          n241 = Select(t=w699, s=w697, f=w698) -> (s? t:f=w696:u16)
                          n242 = Bundle By Name(cluster=w703, "RC Configuration"=w696) -> (w702:T6)
                        }
                        frame 12 {
                          n243 = Scan Value(string=w705, format string="%.1f") -> (value=w706:dbl)  [unwired: 1 in, 1 out]
                          n244 = Bundle By Name(cluster=w708, "AC amplitude [V]"=w706) -> (w707:T6)
                        }
                        frame 13 {
                          n245 = Equal?(x=w716, y="Arduino") -> (x = y?=w713:bool)
                          n246 = Select(t=enum16{"Read Arduino", "Enter manually"}."Read Arduino" ("Temperature Readout"), s=w713, f=enum16{"Read Arduino", "Enter manually"}."Enter manually" ("Temperature Readout")) -> (s? t:f=w710:enum16{"Read Arduino", "Enter manually"})
                          n247 = Bundle By Name(cluster=w718, "Temperature Readout"=w710) -> (w717:T6)
                        }
                        frame 14 {
                          n248 = Scan Value(string=w722, format string="%.1f") -> (value=w723:dbl)  [unwired: 1 in, 1 out]
                          n249 = Bundle By Name(cluster=w721, "Fraction of good strips [%]"=w723) -> (w719:T6)
                        }
                        frame 15 {
                          n250 = Decimal String To Number(string=w726) -> (number=w725:i32)  [unwired: 2 in, 1 out]
                          n251 = Bundle By Name(cluster=w729, "Probe Card Channels"=w725) -> (w727:T6)
                        }
                      }
                    }
                  }
                }
              }
              n252 = call <vilib>:"Close File+.vi"("error in (no error)"=w587, "refnum"=w588) -> ()  [unwired: 3 in, 3 out]
            }
            frame Error {
              n253 = One Button Dialog(message="Can't open definitions file!") -> ()  [unwired: 1 in, 1 out]
            }
          }
          n254 = global write "QC_MeasurementSetup.vi" "Striptest Measurement Parameters"(w578) -> ()
        }
      }
    }
  }
